vi "Read Job.vi"(11 "Jobber Proxy in":refnum<class "Jobber Proxy.lvclass">) -> (2 "Job":refnum<class "Job.lvclass">)   [LabVIEW 2014, in "Jobber Proxy.lvlib" / "Jobber Proxy.lvclass"]
uses:
  Jobber Proxy.lvclass
  Classes/Job/Job.lvclass
  Jobber Proxy.lvclass/Jobber Proxy.ctl
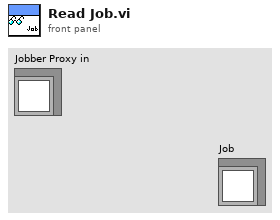
[diagram p1: front panel]
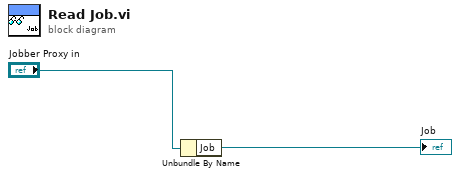
[diagram p0: block diagram]
diagram:
  n1 = Unbundle By Name("Jobber Proxy in") -> ("Job"=→"Job":refnum<class "Job.lvclass">)
